vi "Test_Load-Save_Gasfile.vi"() -> ()   [LabVIEW 2016]
panel:
  out "Saved":bool
  out "Loaded":bool
  in  "Gas_Filename":string="Default"
  in  "Mode (Load)":enum16{"Load", "Save", "SaveAs"}(ring)
  out "Gas_Filepath":path
  in  "Gas Setpoints":T1={"Flow SP (l/min)"=15.0, "F1 N2 (%)"=70.0, "F1 H2 (%)"=0.0, "F1 CO (%)"=10.0, "F1 CO2 (%)"=20.0} {"F1 H2 (%)" min=0.0 max=100.0 format="%.1f"; "F1 CO2 (%)" min=0.0 max=100.0 format="%.1f"; "F1 CO (%)" min=0.0 max=100.0 format="%.1f"; "F1 N2 (%)" min=-10.0 max=100.0 format="%.1f"; "Flow SP (l/min)" min=0.0 max=30.0 format="%.1f"}
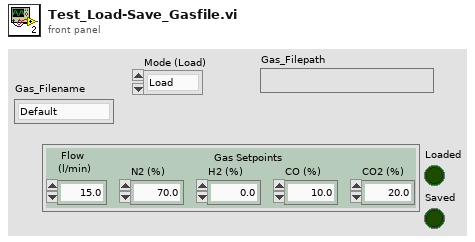
[diagram p1: front panel]
types:
  T1 = cluster{"Flow SP (l/min)":dbl, "F1 N2 (%)":dbl, "F1 H2 (%)":dbl, "F1 CO (%)":dbl, "F1 CO2 (%)":dbl}
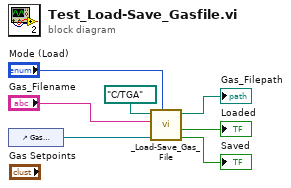
[diagram p0: block diagram]
diagram:
  n1 = control-ref of="Gas Setpoints"() -> (w7:refnum<vi>)
  n2 = call "_Load-Save_Gas_File.vi"("Mode (Load)"="Mode (Load)", "Gas_Setpoints_ref"=w7, "Gas_Filename"="Gas_Filename", "Gas_Folder"=path "C:/TGA") -> ("Saved"=→"Saved":bool, "Loaded"=→"Loaded":bool, "Gas_Filepath"=→"Gas_Filepath":path)  [unwired: 4 in, 1 out]
